vi "Theta Align.vi"(4 "Type":enum16{"Hub", "Corner of Field"}(ring), 6 "Robot Velocities In":T2={"X Velocity"=0.9432032065808408, "Y Velocity"=0.4550691206135685, "Rotational \nVelocity"=-0.0}) -> (2 "Robot Velocities Out":T2={"X Velocity"=0.9432032065808408, "Y Velocity"=0.4550691206135685, "Rotational \nVelocity"=27.751168625617147})   [LabVIEW 2025]
uses:
  swerve-template/Type Definitions/Data/Robot Velocities.ctl
  Framework/Robot Global Data.vi
  <vilib>/addons/control/pid/pid.llb/PID (DBL).vi
  <vilib>/addons/control/pid/NI_PID_pid.lvlib
panel:
  in  "F term":dbl=6.0
  in  "Test angle":dbl=-60.0
  in  "Test with given angle":bool
  out "Pid tuner":cluster{"upper limit":dbl, "upper limit":dbl}(graph)={"upper limit"=35.439177832290056, "upper limit"=43.20648193359375}
  in  "output range":cluster{"output high":dbl, "output low":dbl}={"output high"=300.0, "output low"=-300.0} {"output low" format="%.2f"; "output high" format="%.2f"}
  in  "PID gains":T1={"proportional gain (Kc)"=3.0000000000000004, "integral time (Ti, min)"=0.0, "derivative time (Td, min)"=0.0} {"derivative time (Td, min)" format="%.3f"; "integral time (Ti, min)" format="%.3f"; "proportional gain (Kc)" format="%.3f"}
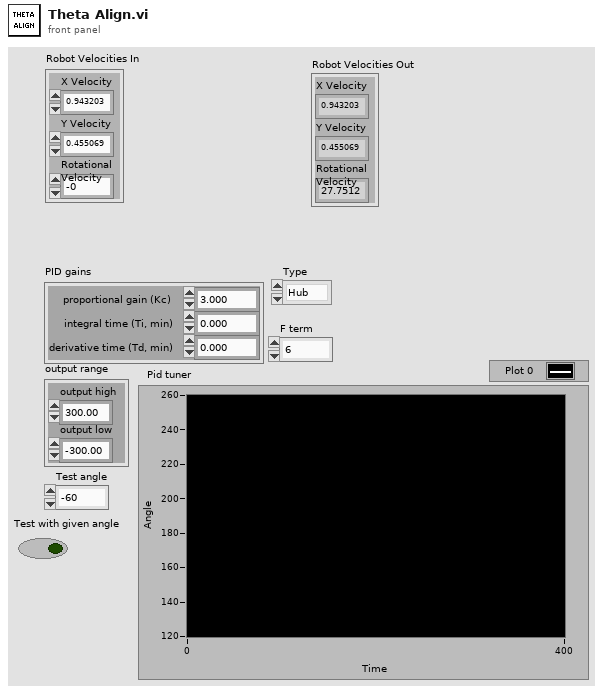
[diagram p1: front panel]
types:
  T1 = cluster{"proportional gain (Kc)":dbl, "integral time (Ti, min)":dbl, "derivative time (Td, min)":dbl}
  T2 = typedef "Robot Velocities.ctl" = cluster{"X Velocity":dbl, "Y Velocity":dbl, "Rotational \nVelocity":dbl}
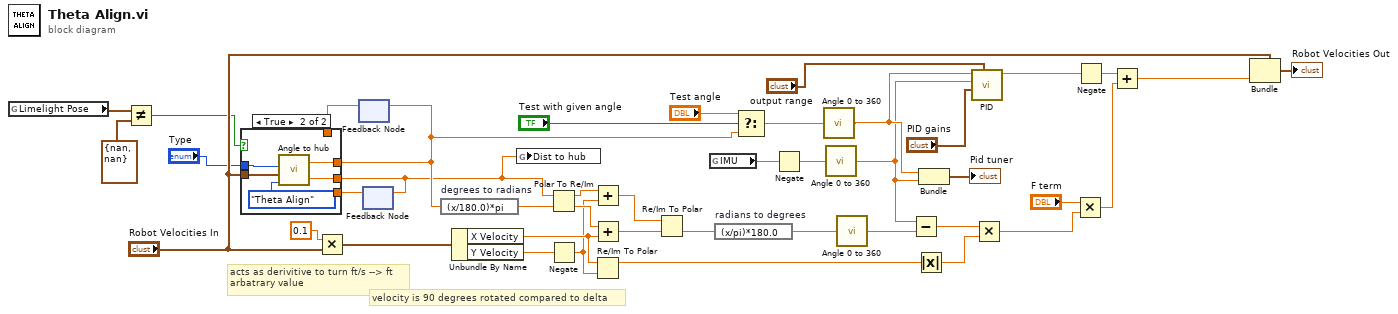
[diagram p0: block diagram]
diagram:
  # "acts as derivitive to turn ft/s --> ft\narbatrary value"
  # "velocity is 90 degrees rotated compared to delta"
  n1 = global read "Robot Global Data.vi" "Limelight Pose"() -> (w3:cluster{"X":dbl, "Y":dbl})
  n2 = Not Equal?(x=w3, y=cluster{"X":dbl, "Y":dbl} {"X"=nan, "Y"=nan}) -> (x != y?=w1:bool)
  n3 = Multiply(x=0.1, y="Robot Velocities In") -> (x*y=w36:T2)
  n4 = feedback #1() -> (w14:dbl)  [unwired: 1 in]
  n5 = feedback #2() -> (w12:dbl)  [unwired: 1 in]
  n6 = case shown="True" w1 {
    tunnel: [w44 w49] -> w15
    tunnel: [w43 w48] -> w13
    tunnel: "Robot Velocities In" -> [_ w46]
    tunnel: w14 -> [w44 _]
    tunnel: w12 -> [w43 _]
    tunnel: "Type" -> [_ w45]
    frame False {
    }
    frame True {
      n7 = call "Angle to hub.vi"("Calculation Mode"=enum16{"Theta Align", "Interp"}."Theta Align", "Robot Velocities In"=w46, "Type"=w45) -> ("Distance to hub"=w48:dbl, "Angle to hub"=w49:dbl)  [unwired: 1 in]
    }
  }
  n8 = feedback-in #1(w15) -> ()
  n9 = feedback-in #2(w13) -> ()
  n10 = expression code="(x/180.0)*pi" "degrees to radians"(w15) -> (w28:dbl)
  n11 = Unbundle By Name(w36) -> ("X Velocity"=w23:dbl, "Y Velocity"=w20:dbl)
  n12 = global write "Robot Global Data.vi" "Dist to hub"(w13) -> ()
  n13 = Polar To Re/Im(2:w28, 3:w13) -> (0:w27:dbl, 1:w22:dbl)
  n14 = Negate(x=w20) -> (-x=w19:dbl)
  n15 = Add(x=w22, y=w19) -> (x+y=w21:dbl)
  n16 = Add(x=w27, y=w23) -> (x+y=w26:dbl)
  n17 = Re/Im To Polar(2:w19, 3:w23) -> (1:w24:dbl)  [unwired: 1 out]
  n18 = Re/Im To Polar(2:w26, 3:w21) -> (0:w7:dbl)  [unwired: 1 out]
  n19 = global read "Robot Global Data.vi" "IMU"() -> (w18:dbl)
  n20 = expression code="(x/pi)*180.0" "radians to degrees"(w7) -> (w6:dbl)
  n21 = Select(t="Test angle", s="Test with given angle", f=w15) -> (s? t:f=w11:dbl)
  n22 = Negate(x=w18) -> (-x=w9:dbl)
  n23 = call "Angle 0 to 360.vi"("Angle in"=w11) -> ("Angle out"=w10:dbl)
  n24 = call "Angle 0 to 360.vi"("Angle in"=w9) -> ("Angle out"=w8:dbl)
  n25 = call "Angle 0 to 360.vi"("Angle in"=w6) -> ("Angle out"=w5:dbl)
  n26 = Subtract(x=w8, y=w5) -> (x-y=w34:dbl)
  n27 = Absolute Value(x=w24) -> (abs(x)=w29:dbl)
  n28 = Bundle("Angle out"=w10, "Angle out"=w8) -> (→"Pid tuner":cluster{"Angle out":dbl, "Angle out":dbl})  [unwired: 1 in]
  n29 = call-poly <vilib>:"PID.vi"("output range"="output range", "PID gains"="PID gains", "process variable"=w8, "setpoint"=w10) -> ("output"=w30:dbl)  [unwired: 6 in, 1 out]
  n30 = Multiply(x=w34, y=w29) -> (x*y=w33:dbl)
  n31 = Multiply(x="F term", y=w33) -> (x*y=w31:dbl)
  n32 = Negate(x=w30) -> (-x=w25:dbl)
  n33 = Add(x=w25, y=w31) -> (x+y=w16:dbl)
  n34 = Bundle(cluster="Robot Velocities In", "Rotational \nVelocity"=w16) -> (→"Robot Velocities Out":T2)  [unwired: 2 in]
